vi "Package Dependencies.vi"(7 "Absolute Paths (F)":bool, 8 "error in (no error)":errorcluster, 11 "NamedPackage in":refnum<class "NamedPackage.lvclass">) -> (0 "error out":errorcluster, 2 "Dependencies":T1[](array[typedef]))   [LabVIEW 2020, in "GPack.lvlib" / "NamedPackage.lvclass"]
uses:
  NamedPackage.lvclass
  Dependency.ctl
  Package Info.ctl
  GPack.lvlib
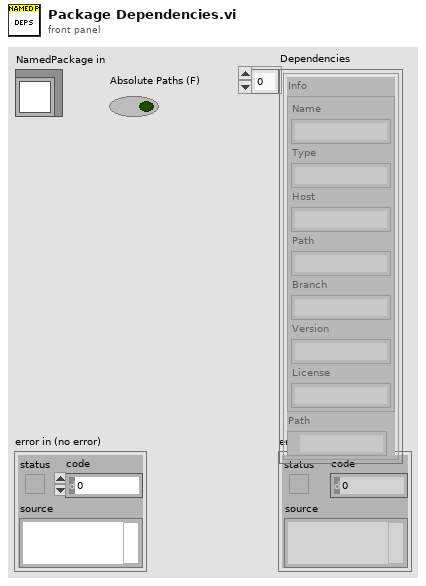
[diagram p1: front panel]
types:
  T1 = typedef "GPack.lvlib/Dependency.ctl" = cluster{"Info":T2, "Path":path}
  T2 = typedef "GPack.lvlib/Package Info.ctl" = cluster{"Name":string, "Type":string, "Host":string, "Path":string, "Branch":string, "Version":string, "License":string}
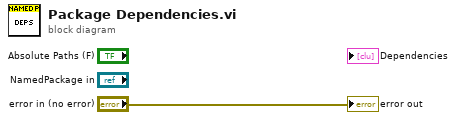
[diagram p0: block diagram]
diagram:
  "error out" <- "error in (no error)"
